vi "Compute Sample Rate.vi"(10 "oversample ratio":dbl=-1.0, 11 "maximum frequency [Hz]":dbl=20000.0) -> (3 "sample rate [Hz]":dbl=nan)   [LabVIEW 2017, in "SV Signal.lvclass"]
doc: "This VI computes a recommended sample rate.\nThis VI will return the requested oversample rate. For oversample rate = -1; This VI will use an oversample rate of 2.5 and will choose the best sample rate from a list of preferred frequencies [51.2k, 102.4k, 204.8k, 2.5*fmax].\n\nThis VI does not prevent the user from selecting a sample rate that violate the Shannon Sampling Theorem (Fs >= 2*F_Nyquist)."
uses:
  <vilib>/addons/_NISVFA/_Generation/Signal Generation/SV Signal/SV Signal.lvclass
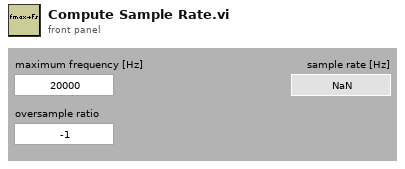
[diagram p1: front panel]
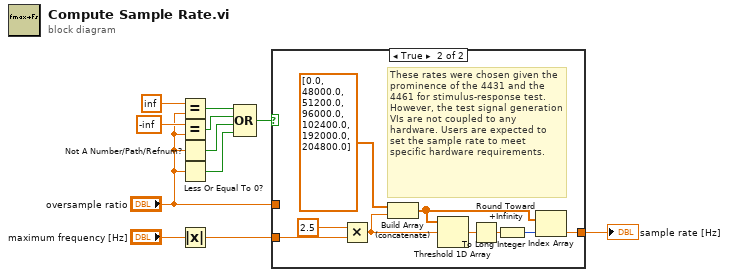
[diagram p0: block diagram]
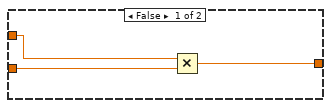
[diagram p2: hidden frame]
diagram:
  n1 = Equal?(x=inf ("y"), y="oversample ratio") -> (x = y?=w6:bool)
  n2 = Equal?(x=-inf ("y"), y="oversample ratio") -> (x = y?=w5:bool)
  n3 = Not A Number/Path/Refnum?(number/path/refnum="oversample ratio") -> (NaN/Path/Refnum?=w3:bool)
  n4 = Less Or Equal To 0?(x="oversample ratio") -> (x <= 0?=w2:bool)
  n5 = Absolute Value(x="maximum frequency [Hz]") -> (abs(x)=w1:dbl)
  n6 = Compound Arithmetic op=OR(w6, w5, w3, w2) -> (w9:bool)
  n7 = case shown="True" w9 {
    tunnel: "oversample ratio" -> [w13 _]
    tunnel: w1 -> [w14 w23]
    tunnel: [w12 w18] -> w7
    frame False {
      n8 = Multiply(x=w13, y=w14) -> (x*y=w12:dbl)
    }
    frame True {
      # "These rates were chosen given the prominence of the 4431 and the 4461 for stimulus-response test. However, the test signal generation VIs are not coupled to any hardware. Users are expected to set the sample rate to meet specific hardware requirements."
      n9 = Multiply(x=2.5 ("y"), y=w23) -> (x*y=w17:dbl)
      n10 = Build Array (concatenate)(dbl[] [0.0, 48000.0, 51200.0, 96000.0, 102400.0, 192000.0, 204800.0], w17) -> (w15:dbl[])
      n11 = Threshold 1D Array(2:w17, 3:w15) -> (0:w21:dbl)  [unwired: 1 in]
      n12 = Round Toward +Infinity(x=w21) -> (ceil(x): smallest int >= x=w20:dbl)
      n13 = To Long Integer(number=w20) -> (32bit integer=w19:i32)
      n14 = Index Array(array=w15, index=w19) -> (element=w18:dbl)
    }
  }
  "sample rate [Hz]" <- w7
